vi "Read.vi"   [LabVIEW 2024, in "Current Value Table.lvlib"]
uses:
  Current Value Table.lvlib
  CVT_DBL/CVT_DBL.lvclass
  CVT_I32/CVT_I32.lvclass
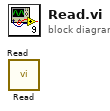
[diagram p0: block diagram]
diagram:
  n1 = call "Read.vi"() -> ()  [unwired: 9 in, 3 out]
  n2 = call "Read.vi"() -> ()  [unwired: 9 in, 3 out]
